vi "fetch_and_translate_trigger.vi"(8 "error in (no error)":errorcluster, 11 "ScanHeadDL090202 in":refnum<class "ScanHeadDL090202.lvclass">) -> (0 "error out":errorcluster, 1 "sender TLC type":T1, 2 "internal trigger":T2, 3 "ScanHeadDL090202 out":refnum<class "ScanHeadDL090202.lvclass">)   [LabVIEW 2010, in "ScanHeadDL090202.lvclass"]
uses:
  ScanHeadDL090202.lvclass
  internal_trigger_enum.ctl
  common/enumerations/top-level_component_type_enum.ctl
  GenericScanHead/GenericScanHead/trigger_enum.ctl
  common/classes/ErrorController/ErrorController/class_data.vi
  GenericScanHead/GenericScanHead/GenericScanHead.lvclass
  common/classes/ErrorController/ErrorController/ErrorController.lvclass
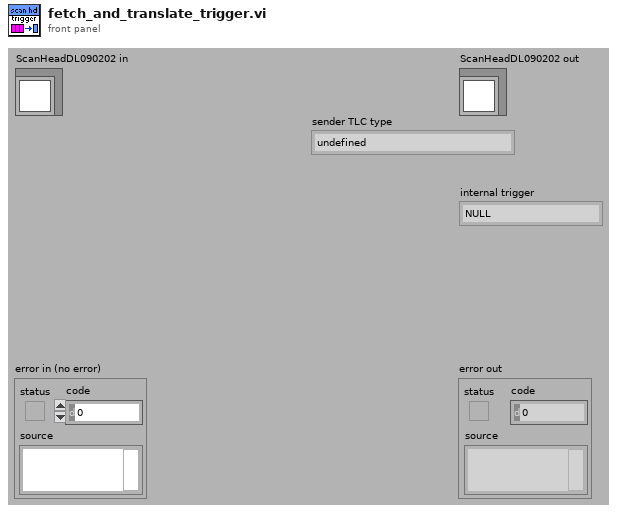
[diagram p1: front panel]
types:
  T1 = typedef "top-level_component_type_enum.ctl" = enum16{"undefined", "ImagingMode", "ScanHead", "DAQ", "ImageAssembler", "Display", "DataCollection", "Analyser", "Stimulator", "ExperimentController", "Instrument", "Stage"}
  T2 = typedef "ScanHeadDL090202.lvclass/internal_trigger_enum.ctl" = enum16{"NULL", "initialise", "terminate", "start scanning", "stop scanning", "scale", "rotate", "tilt", "translate", "update modifiers", "fetch trajectory", "set run mode", "initialise scanners", "terminate scanners", "generate trajectory", "prepare writing", "write", "calculate scanner delays", "fetch position feedback"}
  T3 = typedef "GenericScanHead.lvclass/trigger_enum.ctl" = enum16{"NULL", "fetch trajectory", "generate trajectory", "change run mode", "update modifiers"}
  T4 = typedef "GenericToplevelComponent.lvclass/common_trigger_enum.ctl" = enum16{"NULL", "initialise", "terminate", "fetch command", "fetch data", "attach observer", "register as observer", "detach observer", "acknowledge", "start", "stop", "sweep started", "sweep finished", "experiment started", "experiment stopped"}
  T5 = typedef "trigger_type_enum.ctl" = enum8{"external", "internal", "common"}
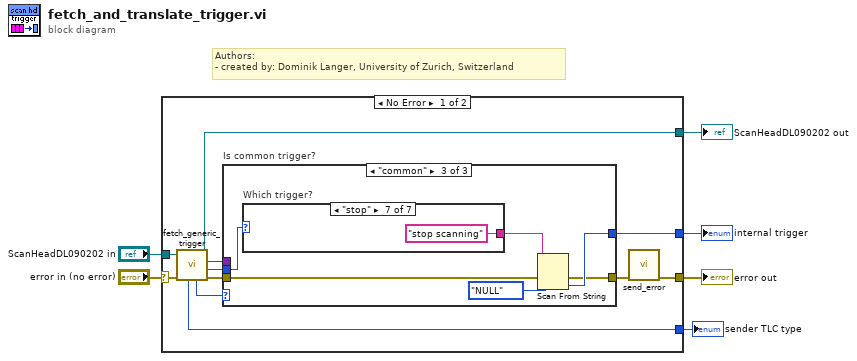
[diagram p0: block diagram]
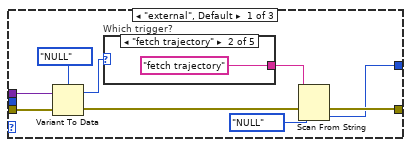
[diagram p2: hidden frame]
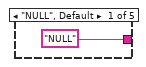
[diagram p3: hidden frame]
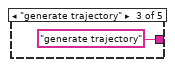
[diagram p4: hidden frame]
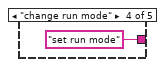
[diagram p5: hidden frame]
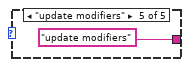
[diagram p6: hidden frame]
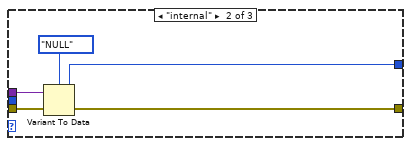
[diagram p7: hidden frame]
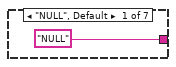
[diagram p8: hidden frame]
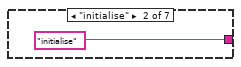
[diagram p9: hidden frame]
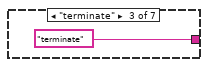
[diagram p10: hidden frame]
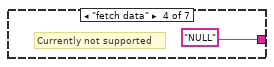
[diagram p11: hidden frame]
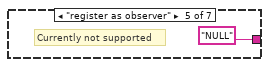
[diagram p12: hidden frame]
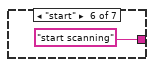
[diagram p13: hidden frame]
diagram:
  # "Authors: \n- created by: Dominik Langer, University of Zurich, Switzerland"
  n1 = case shown="No Error" "error in (no error)" {
    selector: "error in (no error)" -> [w14 w51]
    tunnel: [w16 w51] -> w5
    tunnel: [w11 w50] -> w3
    tunnel: "ScanHeadDL090202 in" -> [w12 w50]
    tunnel: [w17 _] -> w1
    tunnel: [w7 _] -> w2
    frame No Error {
      n2 = call-dynamic "fetch_generic_trigger.vi"("error in (no error)"=w14, "GenericToplevelComponent in"=w12) -> ("error out"=w13:errorcluster, "common trigger"=w8:T4, "trigger"=w9:variant, "GenericToplevelComponent out"=w11:refnum<class "ScanHeadDL090202.lvclass">, "trigger type"=w10:T5, "sender TLC type"=w7:T1)  [unwired: 3 in, 1 out]
      n3 = case "Is common trigger?" shown="\"common\"" w10 {
        tunnel: [w19 w33 w40] -> w17
        tunnel: [w20 w34 w38] -> w15
        tunnel: w13 -> [w23 w35 w39]
        tunnel: w9 -> [w24 w36 _]
        tunnel: w8 -> [_ _ w42]
        frame "external", Default {
          n4 = Variant To Data(error in=w23, Variant=w24, type=trigger_enum."NULL" ("trigger")) -> (error out=w21:errorcluster, data=w26:T3)
          n5 = case "Which trigger?" shown="\"fetch trajectory\"" w26 {
            tunnel: ["NULL" "fetch trajectory" "generate trajectory" "set run mode" "update modifiers"] -> w18
            frame "NULL", Default {
            }
            frame "fetch trajectory" {
            }
            frame "generate trajectory" {
            }
            frame "change run mode" {
            }
            frame "update modifiers" {
            }
          }
          n6 = Scan From String(input string=w18, error in=w21, default 1=internal_trigger_enum."NULL" ("internal trigger")) -> (error out=w20:errorcluster, output 1=w19:T2)  [unwired: 2 in, 2 out]
        }
        frame "internal" {
          n7 = Variant To Data(error in=w35, Variant=w36, type=internal_trigger_enum."NULL" ("internal trigger")) -> (error out=w34:errorcluster, data=w33:T2)
        }
        frame "common" {
          n8 = case "Which trigger?" shown="\"stop\"" w42 {
            tunnel: ["NULL" "initialise" "terminate" "NULL" "NULL" "start scanning" "stop scanning"] -> w37
            frame "NULL", Default {
            }
            frame "initialise" {
            }
            frame "terminate" {
            }
            frame "fetch data" {
              # "Currently not supported"
            }
            frame "register as observer" {
              # "Currently not supported"
            }
            frame "start" {
            }
            frame "stop" {
            }
          }
          n9 = Scan From String(input string=w37, error in=w39, default 1=internal_trigger_enum."NULL" ("internal trigger")) -> (error out=w38:errorcluster, output 1=w40:T2)  [unwired: 2 in, 2 out]
        }
      }
      n10 = call "send_error.vi"("error in (no error)"=w15) -> ("error out"=w16:errorcluster)  [unwired: 10 in]
    }
    frame Error {
    }
  }
  "error out" <- w5
  "ScanHeadDL090202 out" <- w3
  "internal trigger" <- w1
  "sender TLC type" <- w2
